vi "Parse.vi"(8 "error in (no error)":errorcluster, 11 "Transform in":refnum<class "Transform.lvclass">) -> (0 "error out":errorcluster, 3 "Transform out":refnum<class "Transform.lvclass">)   [LabVIEW 2019, in "Transform.lvclass"]
uses:
  Transform.lvclass
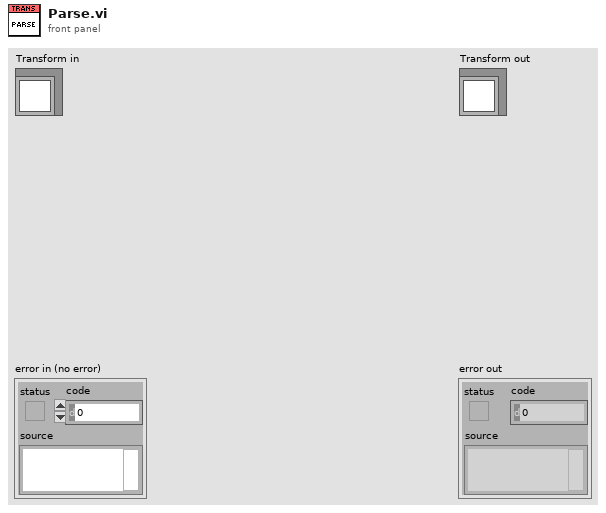
[diagram p1: front panel]
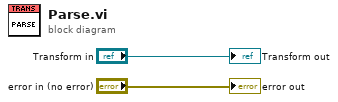
[diagram p0: block diagram]
diagram:
  "error out" <- "error in (no error)"
  "Transform out" <- "Transform in"
